vi "Load Settings on Create.vi"(8 "error in (no error)":errorcluster, 10 "Name":string, 11 "Application in":refnum<class "Application.lvclass">) -> (0 "error out":errorcluster, 2 "Settings":T1, 3 "Application out":refnum<class "Application.lvclass">)   [LabVIEW 2017, in "Application.lvlib" / "Application.lvclass"]
uses:
  Application.lvclass
  Settings/Class Settings -- Cluster.ctl
  <vilib>/TSS/ACRObat Test Framework/Classes/Data/Data Viewer/Settings/Pass Fail Criteria -- Cluster.ctl
  <vilib>/TSS/ACRObat Test Framework/Utilities/Data Persistance/Settings Data/Settings Data.lvclass
  <vilib>/TSS/ACRObat Test Framework/Classes/Data/Data Viewer/Settings/Data Viewer Settings.lvclass
  Settings/App Settings.lvclass
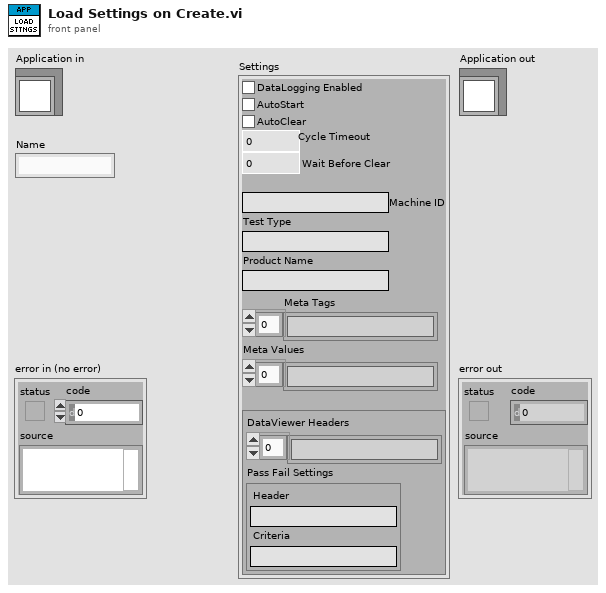
[diagram p1: front panel]
types:
  T1 = typedef "Application.lvlib/App Settings.lvclass/Class Settings -- Cluster.ctl" = cluster{"DataLogging Enabled":bool, "AutoStart":bool, "AutoClear":bool, "Cycle Timeout":u32, "Wait Before Clear":u32, "Machine ID":string, "Test Type":string, "Product Name":string, "Meta Tags":string[], "Meta Values":string[], "Viewer Settings":cluster{"DataViewer Headers":string[], "Pass Fail Settings":T2}}
  T2 = typedef "Data Viewer.lvlib/Data Viewer Settings.lvclass/Pass Fail Criteria -- Cluster.ctl" = cluster{"Header":string, "Criteria":string}
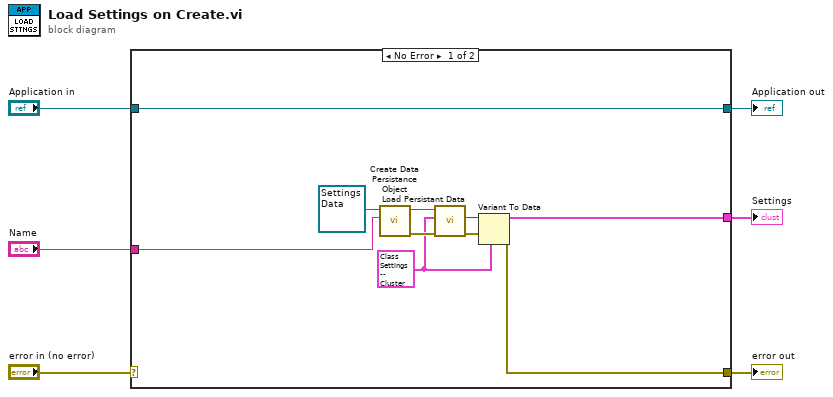
[diagram p0: block diagram]
diagram:
  n1 = case shown="No Error" "error in (no error)" {
    selector: "error in (no error)" -> [_ w18]
    tunnel: [w10 w18] -> w5
    tunnel: [w8 w17] -> w3
    tunnel: "Application in" -> [w8 w17]
    tunnel: [w9 _] -> w2
    tunnel: "Name" -> [w7 _]
    frame No Error {
      w12 = T1 {"DataLogging Enabled"=FALSE, "AutoStart"=FALSE, "AutoClear"=FALSE, "Cycle Timeout"=0, "Wait Before Clear"=0, "Machine ID"="", "Test Type"="", "Product Name"="", "Meta Tags"=[], "Meta Values"=[], "Viewer Settings"={"DataViewer Headers"=[], "Pass Fail Settings"={"Header"="", "Criteria"=""}}} ("Settings")
      n2 = call-dynamic "Create Data Persistance Object.vi"("Object Name"=w7, "Settings Data in"=refnum<class "Settings Data.lvclass"> refnum) -> ("error out"=w16:errorcluster, "Settings Data out"=w14:refnum<class "Settings Data.lvclass">)  [unwired: 8 in]
      n3 = call-dynamic "Load Persistant Data.vi"("error in (no error)"=w16, "Default Data"=w12, "Data Persistance in"=w14) -> ("error out"=w11:errorcluster, "Data"=w13:variant)  [unwired: 6 in, 1 out]
      n4 = Variant To Data(error in=w11, type=w12, Variant=w13) -> (data=w9:T1, error out=w10:errorcluster)
    }
    frame Error {
    }
  }
  "error out" <- w5
  "Application out" <- w3
  "Settings" <- w2
